vi "Equal_Safe_1dI32.vi"(1 "y":i32[](array[numeric]), 2 "x":i32[](array[numeric])) -> (0 "Equal?":bool)   [LabVIEW 2013]
doc: "Checks if arrays x and y are identical (both in length and elements)."
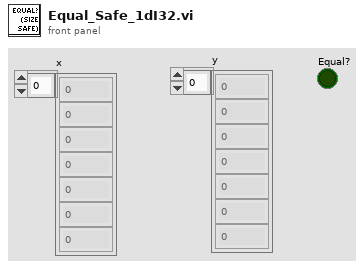
[diagram p1: front panel]
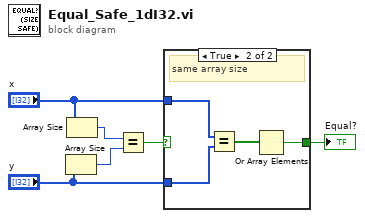
[diagram p0: block diagram]
diagram:
  n1 = Array Size(array="y") -> (size(s)=w5:i32)
  n2 = Array Size(array="x") -> (size(s)=w6:i32)
  n3 = Equal?(x=w6, y=w5) -> (x = y?=w4:bool)
  n4 = case shown="True" w4 {
    selector: w4 -> [w7 _]
    tunnel: "x" -> [_ w11]
    tunnel: "y" -> [_ w10]
    tunnel: [w7 w8] -> w1
    frame False {
      # "different array size"
    }
    frame True {
      # "same array size"
      n5 = Equal?(x=w11, y=w10) -> (x = y?=w9:bool[])
      n6 = Or Array Elements(Boolean array=w9) -> (logical OR=w8:bool)
    }
  }
  "Equal?" <- w1
